vi "Drive Controller.vi"(8 "error in":errorcluster) -> ()   [LabVIEW 2018]
doc: "This VI executes continuously carrying out the current operation and responding to updates or new operation requests. It will often contain the timing or control code that is difficult to place directly in TeleOp. This VI generally opens all sensors and motors and isolates the rest of the robot code from knowing implementation details of how the operations are carried out."
uses:
  <vilib>/Rock Robotics/WPI/Framework/Completion Status.ctl
  Drive Setpoints.ctl
  Drive Operations.ctl
  Support Code/Path Data.ctl
  Support Code/Availible Command systems for auto.ctl
  <vilib>/Rock Robotics/WPI/ThirdParty/REV Robotics/SPARK MAX/Typedef/Spark MAX Control Type.ctl
  <vilib>/Rock Robotics/WPI/RobotDrive/WPI_RobotDriveArcadeDrive_Standard(NoSaturation).vi
  <vilib>/Rock Robotics/Network Tables/NT Read Number.vi
  <vilib>/Rock Robotics/Network Tables/NT Write Number.vi
  <vilib>/Rock Robotics/Network Tables/NT Write Boolean.vi
  ADIS16448 IMU/ADIS16448_IMU.lvlib
panel:
  in  "Time Home":u32=700
  in  "Time 90":u32=1000
  in  "Time 180":u32=1000
  in  "Interactive Values":T1 {"Auto Path Data"."Commands"."System" items=["FLoating Intake"=2, "Carriage Intake"=1, "Elevator"=0]; "Auto Path Data"."Commands"."System Selection" items=["FLoating Intake"=2, "Carriage Intake"=1, "Elevator"=0]}
  in  "Buttons":cluster{"Execute Cmd":bool, "Abort Cmd":bool}
  out "Command Timing":cluster{"Start Time (ms)":u32, "Iterations":i32}
  out "Status":T5
  out "Setpoints":T6(graph)
  out "Current\nCmd":string
  # "Tip: The graph shows the motor setpoints. It may also be helpful to observe inputs and sensor values.\nYou may also want to display tuning or debugging controls."
  # "Interactive Command: You may fill in the settings for a command\nand schedule it with the Execute button. You can observe and abort\nany command while fine tuning the code for the controller."
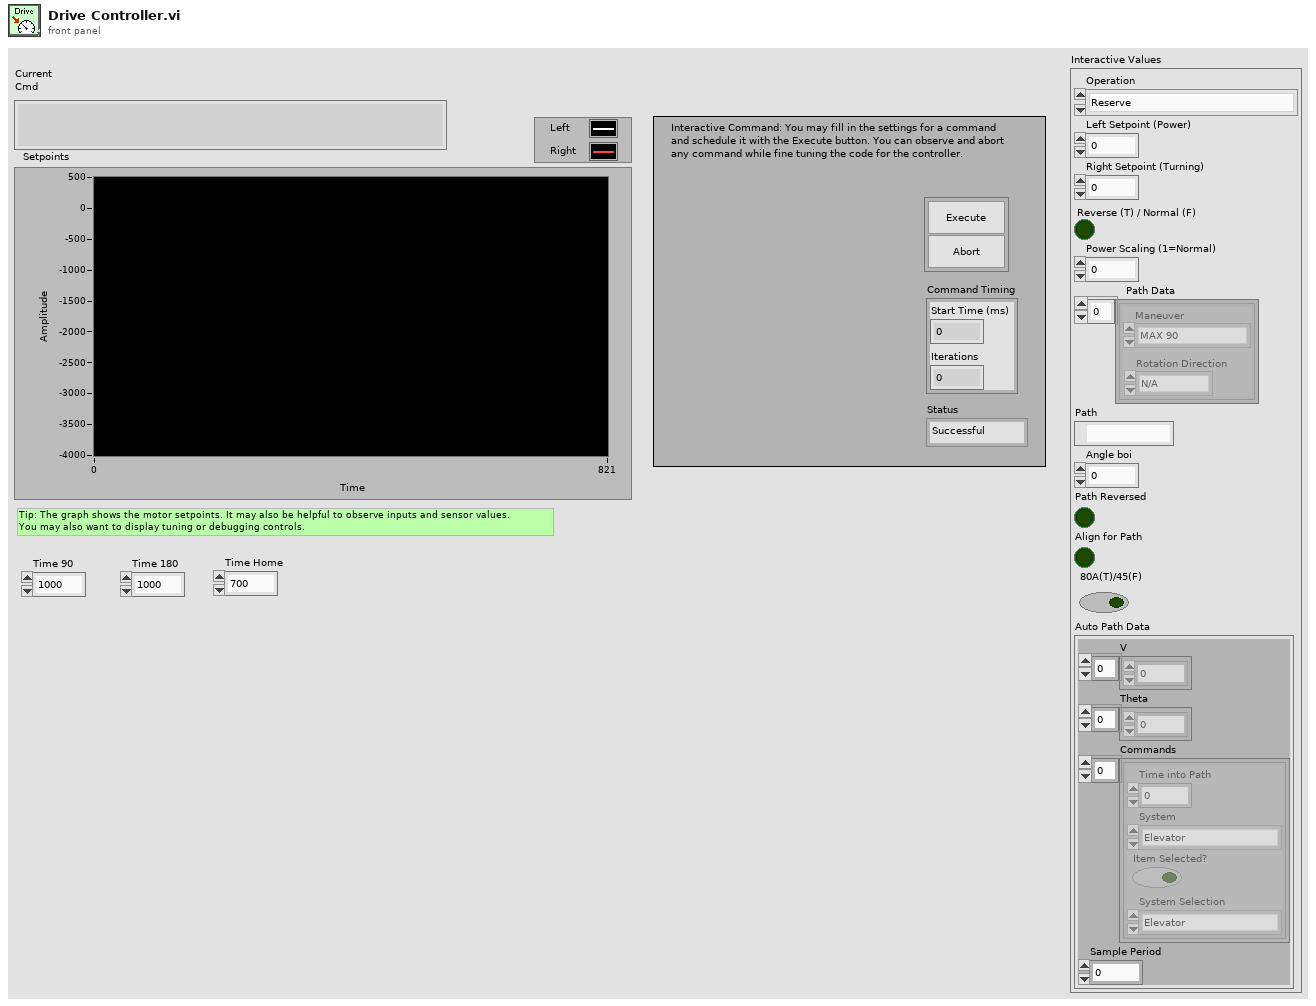
[diagram p1: front panel]
types:
  T1 = typedef "Drive Setpoints.ctl" = cluster{"Operation":T2, "Left Setpoint (Power)":dbl, "Right Setpoint (Turning)":dbl, "Reverse (T) / Normal (F)":bool, "Power Scaling (1=Normal) ":dbl, "Path Data":T3, "Path":path, "Angle boi":dbl, "Path Reversed":bool, "Align for Path":bool, "80A(T)/45(F)":bool, "Auto Path Data":cluster{"V":dbl[], "Theta":dbl[], "Commands":cluster{"Time into Path":dbl, "System":T4, "Item Selected?":bool, "System Selection":T4}[], "Sample Period":dbl}}
  T2 = typedef "Drive Operations.ctl" = enum16{"Reserve", "Read Current", "Immediate", "J-Turn", "Play Back From Log", "Auto-Align"}
  T3 = typedef "Path Data.ctl" = cluster{"Maneuver":enum16{"MAX 90", "MAX 180", "Turn to Home", "Turn to Rocket", "Auto-Align", "Turn to ..."}, "Rotation Direction":enum16{"N/A", "Right", "Left"}}[]
  T4 = typedef "Availible Command systems for auto.ctl" = u16
  T5 = typedef "Completion Status.ctl" = enum16{"Successful", "Aborted", "Incomplete"}
  T6 = cluster{"Left Setpoint":dbl, "Right Setpoint":dbl}
  T7 = cluster{"P Gain":dbl, "I Gain":dbl, "D Gain":dbl, "F Gain":dbl, "I Zone":dbl, "Min Output":dbl, "Max Output":dbl}
  T8 = typedef "WPI_MotorControlDeviceRef.ctl" = cluster{"DeviceStatus":errorcluster, "Type":T9, "PWM":cluster{"PWM Channel":T10, "DeadBand":T11}, "CAN":cluster{"Device Number":u8, "SetOutput VI Ref":variant, "GetOutput VI Ref":variant, "Enable VI Ref":variant, "Disable VI Ref":variant, "Data":variant}, "Invert":bool, "DIO PWM":cluster{"PWM \"Enable\" Channel":T10, "DIOChannel":T12, "PWM Rate":dbl}}
  T9 = typedef "WPI_MotorControlType.ctl" = enum16{"PWM", "CAN", "DIO PWM"}
  T10 = typedef "FPGA_DIOPWMChannel.ctl" = enum8{"PWM 0", "PWM 1", "PWM 2", "PWM 3", "PWM 4", "PWM 5", "PWM 6", "PWM 7", "PWM 8", "PWM 9", "PWM MXP 0", "PWM MXP 1", "PWM MXP 2", "PWM MXP 3", "PWM MXP 4", "PWM MXP 5", "PWM MXP 6", "PWM MXP 7", "PWM MXP 8", "PWM MXP 9", "Invalid"}
  T11 = typedef "WPI_PWMDeadband.ctl" = cluster{"Name":string, "maxPositivePwm":i32, "minPositivePwm":i32, "centerPwm":i32, "maxNegativePwm":i32, "minNegativePwm":i32, "angularRange":u16}
  T12 = typedef "FPGA_DIOChannel.ctl" = enum8{"DIO 0", "DIO 1", "DIO 2", "DIO 3", "DIO 4", "DIO 5", "DIO 6", "DIO 7", "DIO 8", "DIO 9", "DIO MXP 0", "DIO MXP 1", "DIO MXP 2", "DIO MXP 3", "DIO MXP 4", "DIO MXP 5", "DIO MXP 6", "DIO MXP 7", "DIO MXP 8", "DIO MXP 9", "DIO MXP 10", "DIO MXP 11", "DIO MXP 12", "DIO MXP 13", "DIO MXP 14", "DIO MXP 15", "SPI Port CS1", "SPI Port CS2", "SPI Port CS3", "SPI Port MISO", "SPI Port MOSI", "Invalid"}
  T13 = typedef "WPI_RobotDriveDevRef.ctl" = cluster{"DevStatus":errorcluster, "Motors[]":T8[], "Square Inputs":bool, "Max Output":dbl}
  T14 = typedef "ADIS16448_IMU.lvlib/ADI_IMU_ADIS16448_IMUDevRef.ctl" = cluster{"DevStatus":errorcluster, "Handle":i32, "SPI Bus":T15, "Device Found":bool, "Device Ready":bool, "Yaw Axis":enum16{"X", "Y", "Z"}, "AHRS Algorithm":enum16{"Complementary", "Madgwick"}, "Serial":u16, "Lot ID 2":u16, "Lot ID 1":u16, "Bytes Per Sample":u16, "Calibrate On Open?":bool}
  T15 = typedef "spi_bus.ctl" = enum16{"SPI On-Board, CS0", "SPI On-Board, CS1", "SPI On-Board, CS2", "SPI On-Board, CS3", "SPI MXP", "Invalid"}
  T16 = typedef "Command Status Info.ctl" = cluster{"Name":string, "Status":T5, "notifier out":T17}
  T17 = typedef "Completion Notifier.ctl" = refnum<notifier>
  T18 = cluster{"SubSystem Data":T1, cluster{"Start Time (ms)":u32, "Iterations":i32}, cluster{"Command Info":T16, "Description":string, "Default Command":T1, "queue out":refnum<queue>, "Subsystem Name":string}}
  T19 = enum16{"MAX 90", "MAX 180", "Turn to Home", "Turn to Rocket", "Auto-Align"}
  T20 = cluster{"proportional gain (Kc)":dbl, "integral time (Ti, min)":dbl, "derivative time (Td, min)":dbl}
  T21 = cluster{"V":dbl[], "Theta":dbl[], "Commands":cluster{"Time into Path":dbl, "System":T4, "Item Selected?":bool, "System Selection":T4}[], "Sample Period":dbl}
  T22 = cluster{"Maneuver":enum16{"MAX 90", "MAX 180", "Turn to Home", "Turn to Rocket", "Auto-Align", "Turn to ..."}, "Rotation Direction":enum16{"N/A", "Right", "Left"}}
  T23 = enum16{"MAX 90", "MAX 180", "Turn to Home", "Turn to Rocket", "Auto-Align", "Turn to ..."}
  T24 = typedef "Spark MAX Control Type.ctl" = enum16{"Percent VBus", "Voltage", "Velocity", "Position", "Smart Motion", "Current", "Smart Velocity"}
  T25 = cluster{"Time into Path":dbl, "System":T4, "Item Selected?":bool, "System Selection":T4}[]
  T26 = cluster{"Don't move motors while reserved":dbl, "Don't move motors while reserved":dbl}
  T27 = cluster{"SubSystem Data":T1, cluster{"Start Time (ms)":u32, "Iterations":i32}, "Default Command Arguments":cluster{"Command Info":T16, "Description":string, "Default Command":T1, "queue out":refnum<queue>, "Subsystem Name":string}}
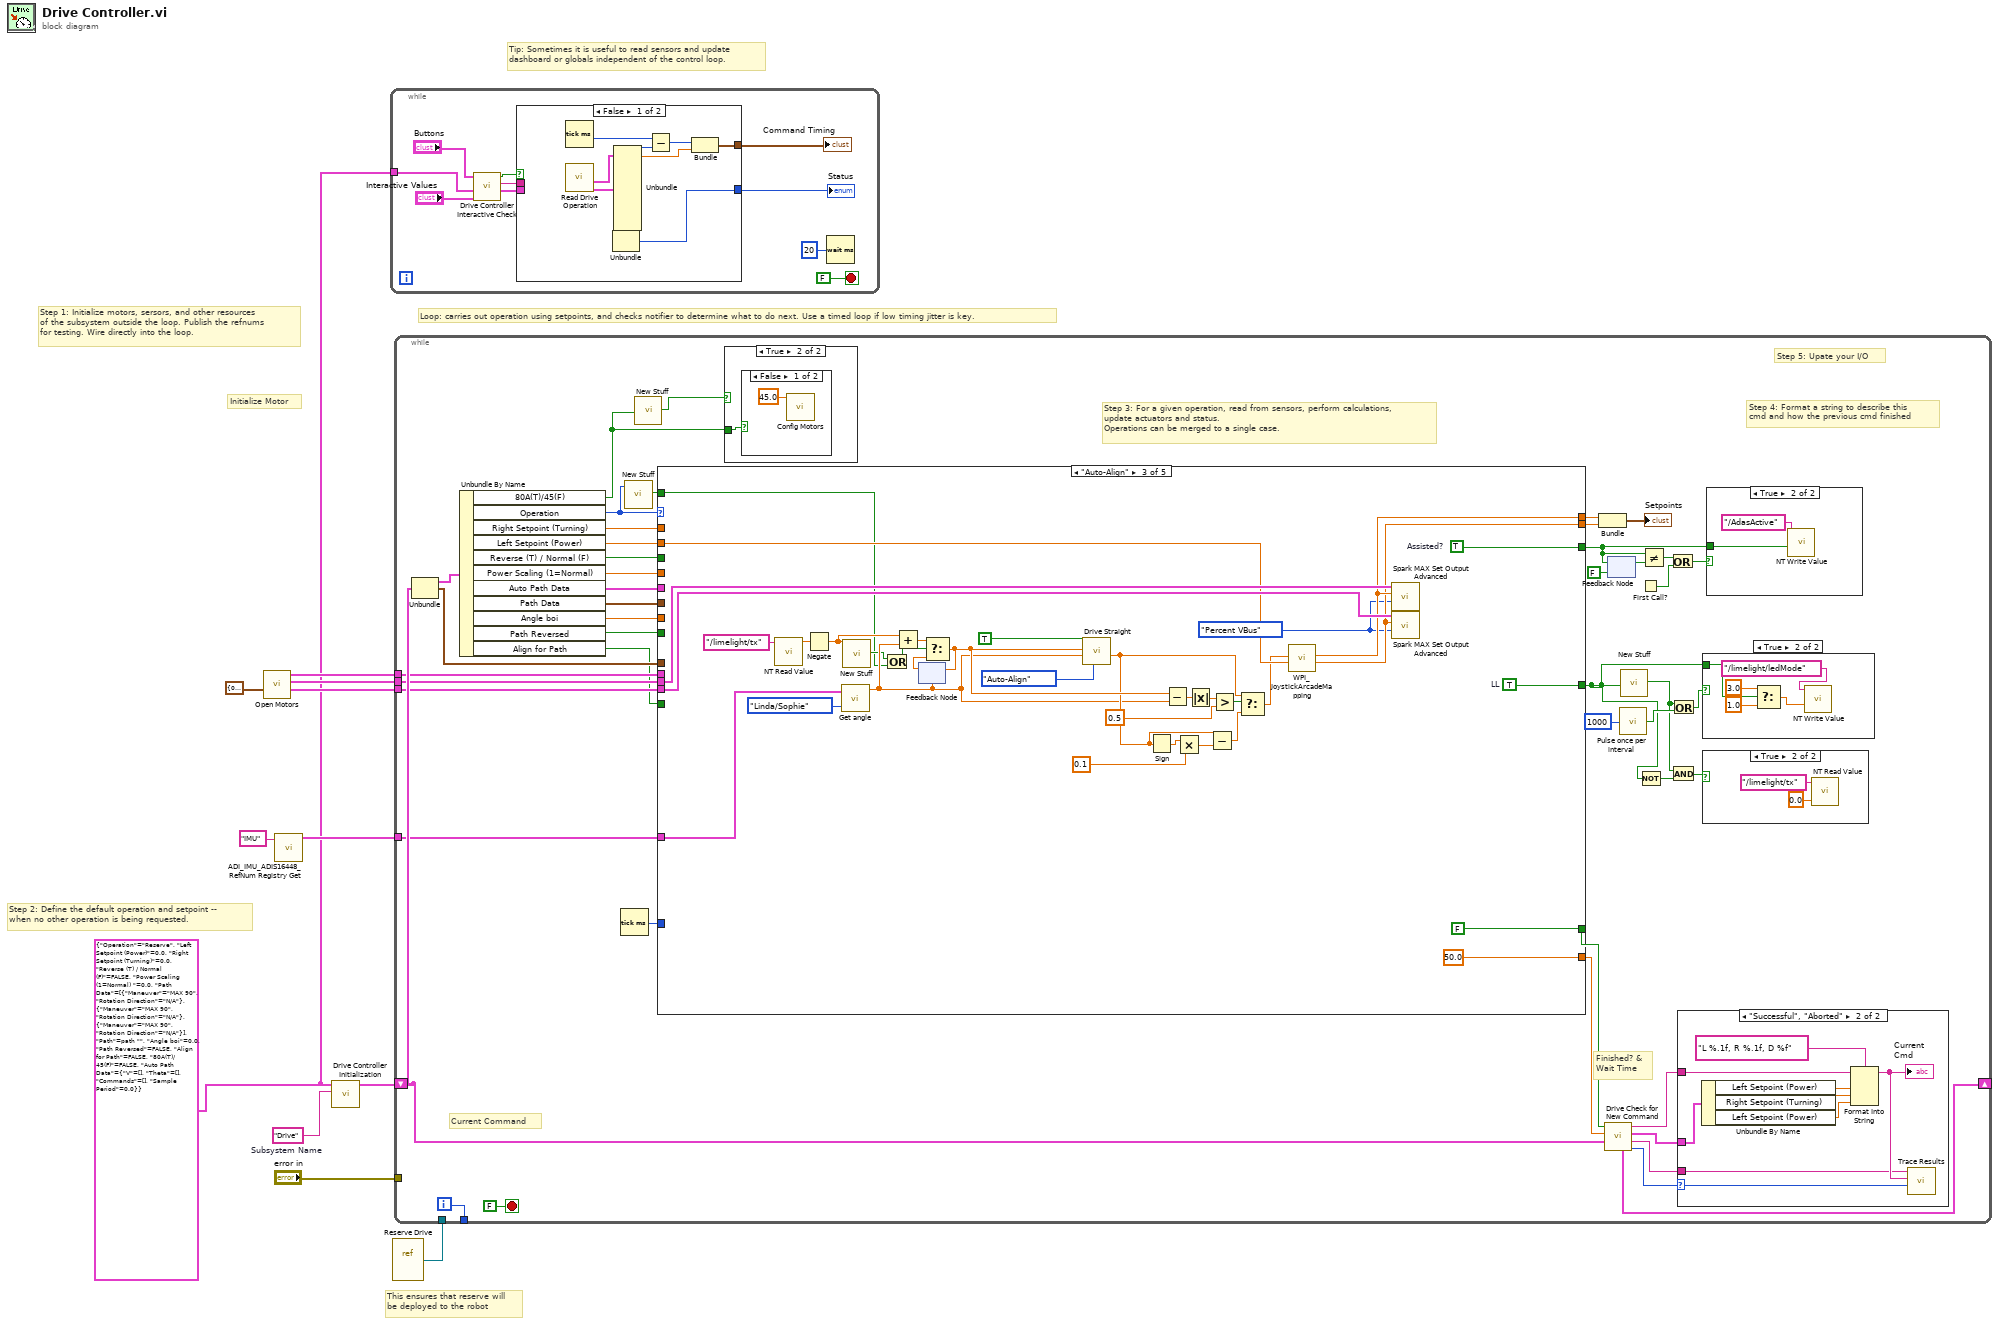
[diagram p0: block diagram]
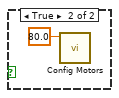
[diagram p4: hidden frame]
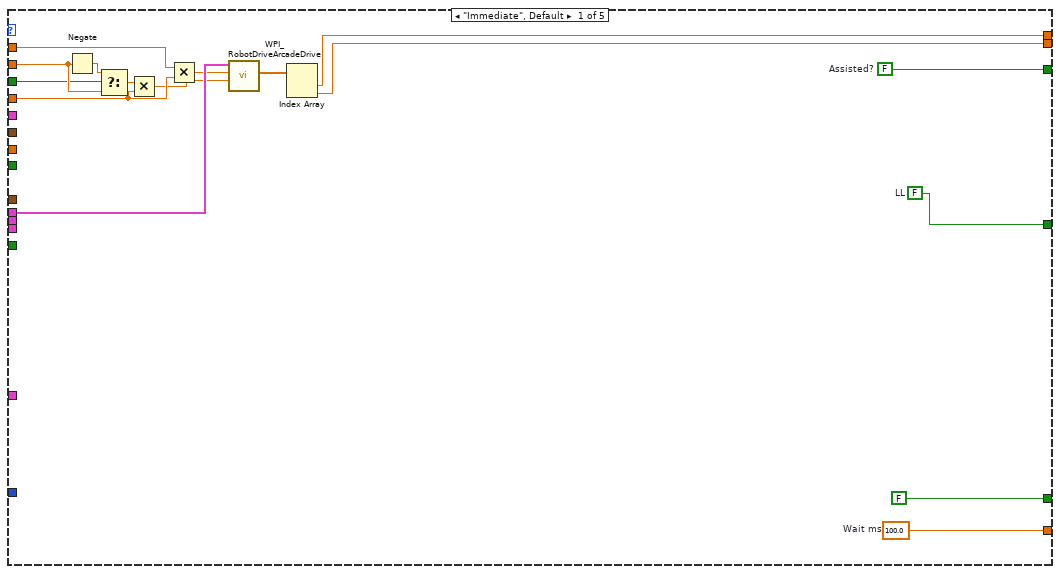
[diagram p6: hidden frame]
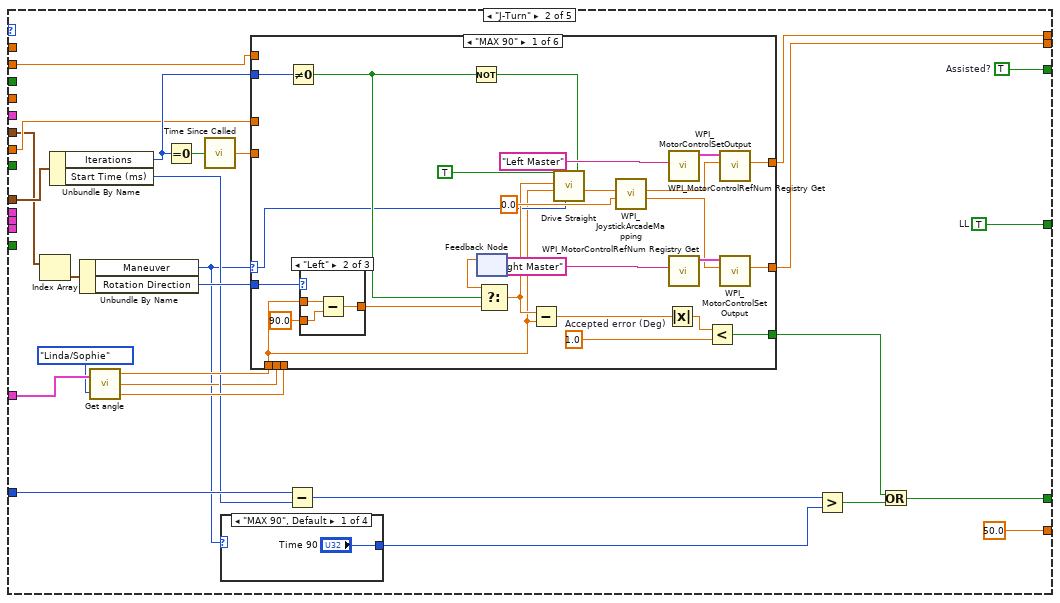
[diagram p7: hidden frame]
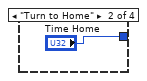
[diagram p8: hidden frame]
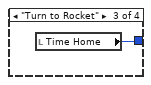
[diagram p9: hidden frame]
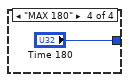
[diagram p10: hidden frame]
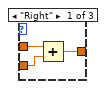
[diagram p11: hidden frame]
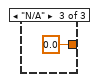
[diagram p12: hidden frame]
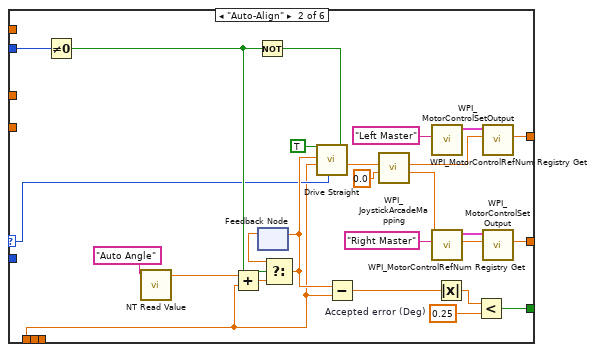
[diagram p13: hidden frame]
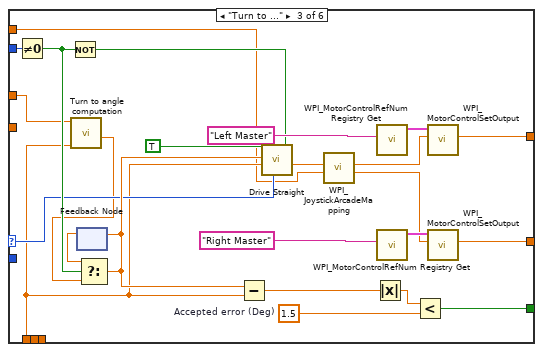
[diagram p14: hidden frame]
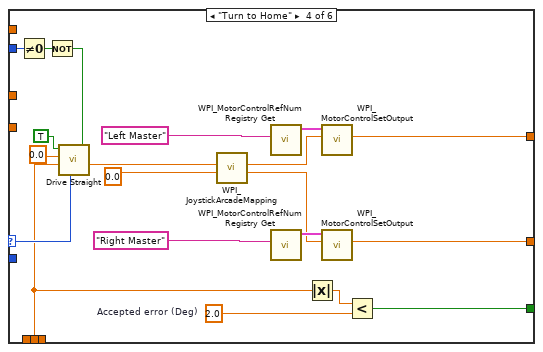
[diagram p15: hidden frame]
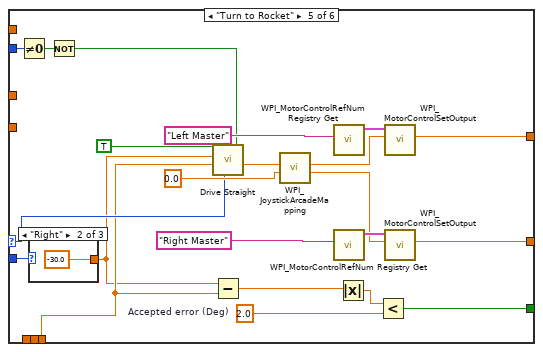
[diagram p16: hidden frame]
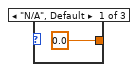
[diagram p17: hidden frame]
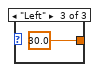
[diagram p18: hidden frame]
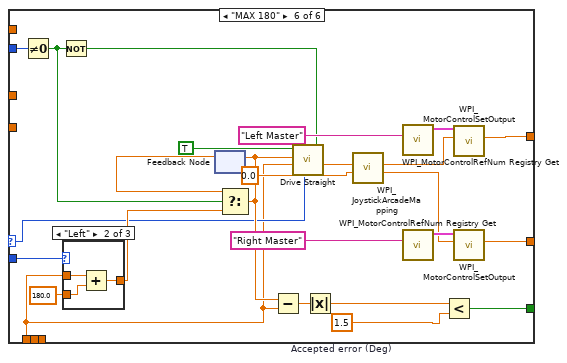
[diagram p19: hidden frame]
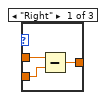
[diagram p20: hidden frame]
diagram:
  w1 = T1 {"Operation"=enum."Reserve", "Left Setpoint (Power)"=0.0, "Right Setpoint (Turning)"=0.0, "Reverse (T) / Normal (F)"=FALSE, "Power Scaling (1=Normal) "=0.0, "Path Data"=[{"Maneuver"=enum."MAX 90", "Rotation Direction"=enum."N/A"}, {"Maneuver"=enum."MAX 90", "Rotation Direction"=enum."N/A"}, {"Maneuver"=enum."MAX 90", "Rotation Direction"=enum."N/A"}], "Path"=path "", "Angle boi"=0.0, "Path Reversed"=FALSE, "Align for Path"=FALSE, "80A(T)/45(F)"=FALSE, "Auto Path Data"={"V"=[], "Theta"=[], "Commands"=[], "Sample Period"=0.0}} ("SubSystem Data")
  w11 = "Drive"  # Subsystem Name
  # "Initialize Motor"
  # "This ensures that reserve will\nbe deployed to the robot"
  # "Tip: Sometimes it is useful to read sensors and update\ndashboard or globals independent of the control loop."
  # "Step 2: Define the default operation and setpoint --\nwhen no other operation is being requested."
  # "Step 1: Initialize motors, sersors, and other resources\nof the subsystem outside the loop. Publish the refnums\nfor testing. Wire directly into the loop."
  # "Loop: carries out operation using setpoints, and checks notifier to determine what to do next. Use a timed loop if low timing jitter is key."
  n1 = call "Open Motors.vi"("PID Constants"=T7 {"P Gain"=0.00035, "I Gain"=5e-07, "D Gain"=0.0, "F Gain"=0.0002, "I Zone"=0.0, "Min Output"=-1.0, "Max Output"=1.0} ("PID Constants for Sparks")) -> ("Right"=w2:T8, "Left"=w3:T8, "WPI Robot"=w4:T13)  [unwired: 7 in, 1 out]
  n2 = call "ADI_IMU_ADIS16448_RefNum Registry Get.vi"("refnum name"="IMU") -> ("ADI IMU DevRef"=w6:T14)  [unwired: 9 in, 1 out]
  n3 = call "Drive Controller Initialization.vi"("Subsystem Name"=w11, "Default Command"=w1) -> ("Current Command"=w9:T18)  [unwired: 9 in]
  n4 = while {
    tunnel: w1 -> [w13]
    stop <- FALSE stop-if-true
    n5 = call "Drive Controller Interactive Check.vi"("Interactive Command In"="Interactive Values", "Default Command"=w13, "Buttons"="Buttons") -> ("Interactive Command Out"=w15:T1, "Trace String"=w16:string, "Schedule"=w17:bool)  [unwired: 6 in]
    n6 = case shown="False" w17 {
      tunnel: [w26 w34] -> w18
      tunnel: [w25 w30] -> w19
      tunnel: w16 -> [_ w32]
      tunnel: w15 -> [_ w31]
      frame False {
        n7 = Tick Count (ms)() -> (millisecond timer value=w29:u32)
        n8 = call "Read Drive Operation.vi"() -> ("Command Info"=w23:T16, "SubSystem Data"=w22:T1)  [unwired: 9 in, 1 out]
        n9 = Unbundle(w23) -> ("Status"=w26:T5)  [unwired: 2 out]
        n10 = Unbundle(w22) -> ("Operation"=w27:T2, "Left Setpoint (Power)"=w24:dbl)  [unwired: 10 out]
        n11 = Subtract(x=w29, y=w27) -> (x-y=w28:u32)
        n12 = Bundle(w28, "Left Setpoint (Power)"=w24) -> (w25:cluster{u32, "Left Setpoint (Power)":dbl})  [unwired: 1 in]
      }
      frame True {
        n13 = call "Drive Command Helper.vi"("Description"=w32, "SubSystem Data"=w31) -> ("Command Info Out"=w33:T16, "Command Timing"=w30:cluster{"Start Time (ms)":u32, "Iterations":i32})  [unwired: 7 in, 1 out]
        n14 = Unbundle(w33) -> ("Status"=w34:T5)  [unwired: 2 out]
      }
    }
    "Status" <- w18
    "Command Timing" <- w19
    n15 = Wait (ms)(milliseconds to wait=u32 20) -> ()  [unwired: 1 out]
  }
  n16 = vi-ref "Reserve Drive.vi"() -> (w8:refnum<vi>)
  n17 = while {
    shift-right: [w70] -> _
    shift-left: w9 -> [w63]
    tunnel: [w79] -> _
    tunnel: "error in" -> [_]
    tunnel: w8 -> [_]
    tunnel: w4 -> [w62]
    tunnel: w6 -> [w47]
    tunnel: w3 -> [w52]
    tunnel: w2 -> [w51]
    i -> [w79]
    stop <- FALSE stop-if-true
    # "Step 4: Format a string to describe this\ncmd and how the previous cmd finished"
    # "Step 5: Upate your I/O"
    # "Current Command"
    # "Finished? &\nWait Time"
    # "Step 3: For a given operation, read from sensors, perform calculations,\nupdate actuators and status.\nOperations can be merged to a single case."
    n18 = Unbundle(w63) -> ("SubSystem Data"=w75:T1, w64:cluster{"Start Time (ms)":u32, "Iterations":i32})  [unwired: 1 out]
    n19 = Unbundle By Name(w75) -> ("80A(T)/45(F)"=w40:bool, "Operation"=w50:T2, "Right Setpoint (Turning)"=w74:dbl, "Left Setpoint (Power)"=w73:dbl, "Reverse (T) / Normal (F)"=w61:bool, "Power Scaling (1=Normal)"=w60:dbl, "Auto Path Data"=w53:T21, "Path Data"=w39:T3, "Angle boi"=w48:dbl, "Path Reversed"=w46:bool, "Align for Path"=w45:bool)
    n20 = Tick Count (ms)() -> (millisecond timer value=w72:u32)
    n21 = call "New Stuff.vi"("Variant 2"=w50) -> ("x != y?"=w49:bool)  [unwired: 26 in]
    n22 = call "New Stuff.vi"("Variant 16"=w40) -> ("x != y?"=w41:bool)  [unwired: 26 in]
    n23 = case shown="\"Auto-Align\"" w50 {
      tunnel: [w106 50.0 ("Infinite") 50.0 ("Infinite") 20.0 ("Infinite") w364] -> w69
      tunnel: [FALSE ("ignore previous (F)") w128 FALSE ("ignore previous (F)") w349 FALSE ("ignore previous (F)")] -> w68
      tunnel: w64 -> [_ w130 _ w355 w363]
      tunnel: [w95 w125 w322 w346 w366] -> w77
      tunnel: [w94 w124 w321 w347 w366] -> w76
      tunnel: w74 -> [w98 _ _ w339 _]
      tunnel: w73 -> [w104 w112 w323 _ _]
      tunnel: w72 -> [_ w126 _ w354 _]
      tunnel: w62 -> [w101 _ _ _ w367]
      tunnel: w61 -> [w100 _ _ w345 _]
      tunnel: w60 -> [w99 _ _ _ _]
      tunnel: w47 -> [_ w123 w328 w352 w361]
      tunnel: [w97 w115 w327 TRUE ("Assisted?") w365] -> w59
      tunnel: w53 -> [_ _ _ w335 _]
      tunnel: w52 -> [_ _ w325 w337 _]
      tunnel: w51 -> [_ _ w324 w336 _]
      tunnel: w49 -> [_ _ w296 _ _]
      tunnel: w48 -> [_ w113 _ _ _]
      tunnel: w46 -> [_ _ _ w343 _]
      tunnel: w45 -> [_ _ _ w340 _]
      tunnel: [w91 w110 w320 w338 w358] -> w36
      tunnel: w39 -> [_ w109 _ _ _]
      frame "Immediate", Default {
        w91 = FALSE  # LL
        w97 = FALSE  # Assisted?
        w106 = 100.0  # Wait ms
        n24 = Negate(x=w104) -> (-x=w105:dbl)
        n25 = Select(t=w105, s=w100, f=w104) -> (s? t:f=w103:dbl)
        n26 = Multiply(x=w103, y=w99) -> (x*y=w93:dbl)
        n27 = Multiply(x=w98, y=w99) -> (x*y=w92:dbl)
        n28 = call-poly <vilib>:"WPI_RobotDriveArcadeDrive.vi"("Y axis value"=w93, "X axis value"=w92, "RobotDriveDevRef"=w101) -> ("Motor Values"=w96:dbl[])  [unwired: 6 in, 2 out]
        n29 = Index Array(array=w96) -> (element #1=w95:dbl, element #2=w94:dbl)  [unwired: 2 in]
      }
      frame "J-Turn" {
        w110 = TRUE  # LL
        w115 = TRUE  # Assisted?
        n30 = Index Array(array=w109) -> (element=w108:T22)  [unwired: 1 in]
        n31 = Unbundle By Name(w130) -> ("Iterations"=w118:i32, "Start Time (ms)"=w117:u32)
        n32 = Unbundle By Name(w108) -> ("Maneuver"=w107:T23, "Rotation Direction"=w132:enum16{"N/A", "Right", "Left"})
        n33 = call "Get angle.vi"("ADI IMU DevRef Out"=w123, "Robot"=enum16{"Linda/Sophie", "Mule"}."Linda/Sophie") -> ("Out"=w122:dbl, "Turn to Home"=w116:dbl, "Wraped Out"=w121:dbl)
        n34 = Equal To 0?(x=w118) -> (x = 0?=w131:bool)
        n35 = call "Time Since Called.vi"("Reset"=w131) -> ("Numeric"=w133:dbl)
        n36 = case shown="\"MAX 90\", Default" w107 {
          tunnel: ["Time 90" "Time Home" w136 "Time 180"] -> w120
          frame "MAX 90", Default {
          }
          frame "Turn to Home" {
          }
          frame "Turn to Rocket" {
            n37 = local read "Time Home"() -> (w136:u32)
          }
          frame "MAX 180" {
          }
        }
        n38 = case shown="\"MAX 90\"" w107 {
          selector: w107 -> [w140 w174 w199 w222 w243 w272]
          tunnel: [w142 w176 w201 w224 w245 w278] -> w119
          tunnel: w133 -> [_ _ _ _ _ _]
          tunnel: [w150 w184 w209 w230 w251 w269] -> w125
          tunnel: [w147 w181 w206 w227 w248 w266] -> w124
          tunnel: w132 -> [w138 _ _ _ w239 w264]
          tunnel: w118 -> [w141 w175 w200 w223 w244 w276]
          tunnel: w122 -> [w139 w170 w196 _ _ w265]
          tunnel: w121 -> [_ _ _ _ w241 _]
          tunnel: w116 -> [_ _ _ w221 _ _]
          tunnel: w113 -> [_ _ w198 _ _ _]
          tunnel: w112 -> [_ _ w195 _ _ _]
          frame "MAX 90" {
            w154 = 1.0  # Accepted error (Deg)
            n39 = Not Equal To 0?(x=w141) -> (x != 0?=w144:bool)
            n40 = case shown="\"Left\"" w138 {
              tunnel: 90.0 -> [w165 w168 _]
              tunnel: [w164 w167 0.0] -> w161
              tunnel: w139 -> [w163 w166 _]
              frame "Right" {
                n41 = Add(x=w163, y=w165) -> (x+y=w164:dbl)
              }
              frame "Left" {
                n42 = Subtract(x=w166, y=w168) -> (x-y=w167:dbl)
              }
              frame "N/A" {
              }
            }
            n43 = Not(x=w144) -> (.not. x?=w145:bool)
            n44 = feedback #1() -> (w160:dbl)  [unwired: 1 in]
            n45 = Select(t=w160, s=w144, f=w161) -> (s? t:f=w146:dbl)
            n46 = feedback-in #1(w146) -> ()
            n47 = Subtract(x=w146, y=w139) -> (x-y=w143:dbl)
            n48 = call "Drive Straight.vi"("reinitialize? (F)"=w145, "Maneuver"=w140, "Angle"=w139, "Angle to Get"=w146, "Enable?"=TRUE ("Drive Straight?")) -> ("Turn Setpoint"=w157:dbl)  [unwired: 4 in]
            n49 = call <vilib>:"WPI_JoystickArcadeMapping.vi"("Y axis value"=0.0, "X axis value"=w157) -> ("Right Motor Value"=w148:dbl, "Left Motor Value"=w152:dbl)  [unwired: 8 in]
            n50 = Absolute Value(x=w143) -> (abs(x)=w155:dbl)
            n51 = call <vilib>:"WPI_MotorControlRefNum Registry Get.vi"("refnum name"="Left Master") -> ("MotorControlDevRef"=w151:T8)  [unwired: 9 in, 1 out]
            n52 = call <vilib>:"WPI_MotorControlRefNum Registry Get.vi"("refnum name"="Right Master") -> ("MotorControlDevRef"=w149:T8)  [unwired: 9 in, 1 out]
            n53 = Less?(x=w155, y=w154) -> (x < y?=w142:bool)
            n54 = call <vilib>:"WPI_MotorControlSetOutput.vi"("Output"=w152, "MotorControlDevRef"=w151) -> ("Motor Output"=w150:dbl)  [unwired: 7 in, 2 out]
            n55 = call <vilib>:"WPI_MotorControlSetOutput.vi"("Output"=w148, "MotorControlDevRef"=w149) -> ("Motor Output"=w147:dbl)  [unwired: 7 in, 2 out]
          }
          frame "Auto-Align" {
            w188 = 0.25  # Accepted error (Deg)
            n56 = Not Equal To 0?(x=w175) -> (x != 0?=w178:bool)
            n57 = call-poly <vilib>:"NT Read Value.vi"("Name"="Auto Angle") -> ("Numeric"=w171:dbl)  [unwired: 9 in, 1 out]
            n58 = Add(x=w171, y=w170) -> (x+y=w172:dbl)
            n59 = Not(x=w178) -> (.not. x?=w179:bool)
            n60 = feedback #2() -> (w194:dbl)  [unwired: 1 in]
            n61 = Select(t=w194, s=w178, f=w172) -> (s? t:f=w180:dbl)
            n62 = feedback-in #2(w180) -> ()
            n63 = call "Drive Straight.vi"("reinitialize? (F)"=w179, "Maneuver"=w174, "Angle"=w170, "Angle to Get"=w180, "Enable?"=TRUE ("Drive Straight?")) -> ("Turn Setpoint"=w191:dbl)  [unwired: 4 in]
            n64 = Subtract(x=w180, y=w170) -> (x-y=w177:dbl)
            n65 = call <vilib>:"WPI_JoystickArcadeMapping.vi"("Y axis value"=0.0, "X axis value"=w191) -> ("Right Motor Value"=w182:dbl, "Left Motor Value"=w186:dbl)  [unwired: 8 in]
            n66 = call <vilib>:"WPI_MotorControlRefNum Registry Get.vi"("refnum name"="Left Master") -> ("MotorControlDevRef"=w185:T8)  [unwired: 9 in, 1 out]
            n67 = call <vilib>:"WPI_MotorControlRefNum Registry Get.vi"("refnum name"="Right Master") -> ("MotorControlDevRef"=w183:T8)  [unwired: 9 in, 1 out]
            n68 = Absolute Value(x=w177) -> (abs(x)=w189:dbl)
            n69 = Less?(x=w189, y=w188) -> (x < y?=w176:bool)
            n70 = call <vilib>:"WPI_MotorControlSetOutput.vi"("Output"=w186, "MotorControlDevRef"=w185) -> ("Motor Output"=w184:dbl)  [unwired: 7 in, 2 out]
            n71 = call <vilib>:"WPI_MotorControlSetOutput.vi"("Output"=w182, "MotorControlDevRef"=w183) -> ("Motor Output"=w181:dbl)  [unwired: 7 in, 2 out]
          }
          frame "Turn to ..." {
            w213 = 1.5  # Accepted error (Deg)
            n72 = Not Equal To 0?(x=w200) -> (x != 0?=w203:bool)
            n73 = Not(x=w203) -> (.not. x?=w204:bool)
            n74 = call "Turn to angle computation.vi"("Current Angle"=w196, "Angle To Get"=w198) -> ("Current Angle 2"=w197:dbl)  [unwired: 9 in]
            n75 = feedback #3() -> (w218:dbl)  [unwired: 1 in]
            n76 = Select(t=w218, s=w203, f=w197) -> (s? t:f=w205:dbl)
            n77 = feedback-in #3(w205) -> ()
            n78 = Subtract(x=w205, y=w196) -> (x-y=w202:dbl)
            n79 = call "Drive Straight.vi"("reinitialize? (F)"=w204, "Maneuver"=w199, "Angle"=w196, "Angle to Get"=w205, "Enable?"=TRUE ("Drive Straight?")) -> ("Turn Setpoint"=w215:dbl)  [unwired: 4 in]
            n80 = call <vilib>:"WPI_JoystickArcadeMapping.vi"("Y axis value"=w195, "X axis value"=w215) -> ("Right Motor Value"=w207:dbl, "Left Motor Value"=w211:dbl)  [unwired: 8 in]
            n81 = Absolute Value(x=w202) -> (abs(x)=w214:dbl)
            n82 = call <vilib>:"WPI_MotorControlRefNum Registry Get.vi"("refnum name"="Left Master") -> ("MotorControlDevRef"=w210:T8)  [unwired: 9 in, 1 out]
            n83 = call <vilib>:"WPI_MotorControlRefNum Registry Get.vi"("refnum name"="Right Master") -> ("MotorControlDevRef"=w208:T8)  [unwired: 9 in, 1 out]
            n84 = Less?(x=w214, y=w213) -> (x < y?=w201:bool)
            n85 = call <vilib>:"WPI_MotorControlSetOutput.vi"("Output"=w211, "MotorControlDevRef"=w210) -> ("Motor Output"=w209:dbl)  [unwired: 7 in, 2 out]
            n86 = call <vilib>:"WPI_MotorControlSetOutput.vi"("Output"=w207, "MotorControlDevRef"=w208) -> ("Motor Output"=w206:dbl)  [unwired: 7 in, 2 out]
          }
          frame "Turn to Home" {
            w233 = 2.0  # Accepted error (Deg)
            n87 = Not Equal To 0?(x=w223) -> (x != 0?=w225:bool)
            n88 = Not(x=w225) -> (.not. x?=w226:bool)
            n89 = call "Drive Straight.vi"("reinitialize? (F)"=w226, "Maneuver"=w222, "Angle"=w221, "Angle to Get"=0.0 ("Drive Setpoint"), "Enable?"=TRUE ("Drive Straight?")) -> ("Turn Setpoint"=w236:dbl)  [unwired: 4 in]
            n90 = call <vilib>:"WPI_JoystickArcadeMapping.vi"("Y axis value"=0.0, "X axis value"=w236) -> ("Right Motor Value"=w228:dbl, "Left Motor Value"=w232:dbl)  [unwired: 8 in]
            n91 = call <vilib>:"WPI_MotorControlRefNum Registry Get.vi"("refnum name"="Left Master") -> ("MotorControlDevRef"=w231:T8)  [unwired: 9 in, 1 out]
            n92 = call <vilib>:"WPI_MotorControlRefNum Registry Get.vi"("refnum name"="Right Master") -> ("MotorControlDevRef"=w229:T8)  [unwired: 9 in, 1 out]
            n93 = Absolute Value(x=w221) -> (abs(x)=w234:dbl)
            n94 = call <vilib>:"WPI_MotorControlSetOutput.vi"("Output"=w232, "MotorControlDevRef"=w231) -> ("Motor Output"=w230:dbl)  [unwired: 7 in, 2 out]
            n95 = call <vilib>:"WPI_MotorControlSetOutput.vi"("Output"=w228, "MotorControlDevRef"=w229) -> ("Motor Output"=w227:dbl)  [unwired: 7 in, 2 out]
            n96 = Less?(x=w234, y=w233) -> (x < y?=w224:bool)
          }
          frame "Turn to Rocket" {
            w255 = 2.0  # Accepted error (Deg)
            n97 = Not Equal To 0?(x=w244) -> (x != 0?=w246:bool)
            n98 = case shown="\"Right\"" w239 {
              tunnel: [0.0 -30.0 30.0] -> w240
              frame "N/A", Default {
              }
              frame "Right" {
              }
              frame "Left" {
              }
            }
            n99 = Not(x=w246) -> (.not. x?=w247:bool)
            n100 = call "Drive Straight.vi"("reinitialize? (F)"=w247, "Maneuver"=w243, "Angle"=w241, "Angle to Get"=w240, "Enable?"=TRUE ("Drive Straight?")) -> ("Turn Setpoint"=w258:dbl)  [unwired: 4 in]
            n101 = Subtract(x=w240, y=w241) -> (x-y=w242:dbl)
            n102 = call <vilib>:"WPI_JoystickArcadeMapping.vi"("Y axis value"=0.0, "X axis value"=w258) -> ("Right Motor Value"=w249:dbl, "Left Motor Value"=w253:dbl)  [unwired: 8 in]
            n103 = call <vilib>:"WPI_MotorControlRefNum Registry Get.vi"("refnum name"="Left Master") -> ("MotorControlDevRef"=w252:T8)  [unwired: 9 in, 1 out]
            n104 = call <vilib>:"WPI_MotorControlRefNum Registry Get.vi"("refnum name"="Right Master") -> ("MotorControlDevRef"=w250:T8)  [unwired: 9 in, 1 out]
            n105 = Absolute Value(x=w242) -> (abs(x)=w256:dbl)
            n106 = Less?(x=w256, y=w255) -> (x < y?=w245:bool)
            n107 = call <vilib>:"WPI_MotorControlSetOutput.vi"("Output"=w253, "MotorControlDevRef"=w252) -> ("Motor Output"=w251:dbl)  [unwired: 7 in, 2 out]
            n108 = call <vilib>:"WPI_MotorControlSetOutput.vi"("Output"=w249, "MotorControlDevRef"=w250) -> ("Motor Output"=w248:dbl)  [unwired: 7 in, 2 out]
          }
          frame "MAX 180" {
            w279 = 1.5  # Accepted error (Deg)
            n109 = Not Equal To 0?(x=w276) -> (x != 0?=w275:bool)
            n110 = Not(x=w275) -> (.not. x?=w274:bool)
            n111 = case shown="\"Left\"" w264 {
              tunnel: 180.0 -> [w291 w294 _]
              tunnel: [w290 w293 0.0] -> w287
              tunnel: w265 -> [w289 w292 _]
              frame "Right" {
                n112 = Subtract(x=w289, y=w291) -> (x-y=w290:dbl)
              }
              frame "Left" {
                n113 = Add(x=w292, y=w294) -> (x+y=w293:dbl)
              }
              frame "N/A" {
              }
            }
            n114 = feedback #4() -> (w286:dbl)  [unwired: 1 in]
            n115 = Select(t=w286, s=w275, f=w287) -> (s? t:f=w277:dbl)
            n116 = feedback-in #4(w277) -> ()
            n117 = Subtract(x=w277, y=w265) -> (x-y=w281:dbl)
            n118 = call "Drive Straight.vi"("reinitialize? (F)"=w274, "Maneuver"=w272, "Angle"=w265, "Angle to Get"=w277, "Enable?"=TRUE) -> ("Turn Setpoint"=w283:dbl)  [unwired: 4 in]
            n119 = Absolute Value(x=w281) -> (abs(x)=w280:dbl)
            n120 = call <vilib>:"WPI_JoystickArcadeMapping.vi"("Y axis value"=0.0, "X axis value"=w283) -> ("Right Motor Value"=w267:dbl, "Left Motor Value"=w270:dbl)  [unwired: 8 in]
            n121 = call <vilib>:"WPI_MotorControlRefNum Registry Get.vi"("refnum name"="Left Master") -> ("MotorControlDevRef"=w271:T8)  [unwired: 9 in, 1 out]
            n122 = call <vilib>:"WPI_MotorControlRefNum Registry Get.vi"("refnum name"="Right Master") -> ("MotorControlDevRef"=w268:T8)  [unwired: 9 in, 1 out]
            n123 = Less?(x=w280, y=w279) -> (x < y?=w278:bool)
            n124 = call <vilib>:"WPI_MotorControlSetOutput.vi"("Output"=w270, "MotorControlDevRef"=w271) -> ("Motor Output"=w269:dbl)  [unwired: 7 in, 2 out]
            n125 = call <vilib>:"WPI_MotorControlSetOutput.vi"("Output"=w267, "MotorControlDevRef"=w268) -> ("Motor Output"=w266:dbl)  [unwired: 7 in, 2 out]
          }
        }
        n126 = Subtract(x=w126, y=w117) -> (x-y=w129:u32)
        n127 = Greater?(x=w129, y=w120) -> (0:w111:bool)
        n128 = Or(x=w119, y=w111) -> (x .or. y?=w128:bool)
      }
      frame "Auto-Align" {
        w318 = Spark_MAX_Control_Type."Percent VBus" ("Control Mode")
        w320 = TRUE  # LL
        w327 = TRUE  # Assisted?
        n129 = call-poly <vilib>:"NT Read Value.vi"("Name"="/limelight/tx") -> ("Numeric"=w307:dbl)  [unwired: 9 in, 1 out]
        n130 = Negate(x=w307) -> (-x=w306:dbl)
        n131 = call "Get angle.vi"("ADI IMU DevRef Out"=w328, "Robot"=enum16{"Linda/Sophie", "Mule"}."Linda/Sophie") -> ("Out"=w299:dbl)  [unwired: 2 out]
        n132 = call "New Stuff.vi"("Variant"=w306) -> ("x != y?"=w297:bool)  [unwired: 26 in]
        n133 = Or(x=w297, y=w296) -> (x .or. y?=w298:bool)
        n134 = Add(x=w306, y=w299) -> (x+y=w314:dbl)
        n135 = feedback #5(w299) -> (w315:dbl)
        n136 = Select(t=w314, s=w298, f=w315) -> (s? t:f=w309:dbl)
        n137 = feedback-in #5(w309) -> ()
        n138 = call "Drive Straight.vi"("Maneuver"=T19."Auto-Align", "Angle"=w299, "Angle to Get"=w309, "Enable?"=TRUE ("Drive Straight?")) -> ("Turn Setpoint"=w302:dbl)  [unwired: 5 in]
        n139 = Sign(1:w302) -> (0:w304:dbl)
        n140 = Subtract(x=w309, y=w299) -> (x-y=w310:dbl)
        n141 = Multiply(x=w304, y=0.1) -> (x*y=w301:dbl)
        n142 = Absolute Value(x=w310) -> (abs(x)=w311:dbl)
        n143 = Subtract(x=w302, y=w301) -> (x-y=w300:dbl)
        n144 = Greater?(x=w311, y=0.5) -> (0:w312:bool)
        n145 = Select(t=w302, s=w312, f=w300) -> (s? t:f=w308:dbl)
        n146 = call <vilib>:"WPI_JoystickArcadeMapping.vi"("Y axis value"=w323, "X axis value"=w308) -> ("Right Motor Value"=w321:dbl, "Left Motor Value"=w322:dbl)  [unwired: 8 in]
        n147 = call <vilib>:"Spark MAX Set Output Advanced.vi"("Control Mode"=w318, "Setpoint"=w322, "MotorControlDevRef"=w325) -> ()  [unwired: 7 in, 2 out]
        n148 = call <vilib>:"Spark MAX Set Output Advanced.vi"("Control Mode"=w318, "Setpoint"=w321, "MotorControlDevRef"=w324) -> ()  [unwired: 7 in, 2 out]
      }
      frame "Play Back From Log" {
        w338 = TRUE  # LL
        w348 = Spark_MAX_Control_Type."Velocity" ("Control Mode")
        n149 = Unbundle By Name(w355) -> ("Iterations"=w330:i32)
        n150 = Unbundle(w335) -> ("V"=w334:dbl[], "Theta"=w333:dbl[], "Commands"=w332:T25, "Sample Period"=w331:dbl)
        n151 = call "Execute Path with commands.vi"("Iterations"=w330, "Sample Period"=w331, "Commands"=w332) -> ()
        n152 = call "Get angle.vi"("ADI IMU DevRef Out"=w352, "Robot"=enum16{"Linda/Sophie", "Mule"}."Linda/Sophie") -> ("Out"=w351:dbl)  [unwired: 2 out]
        n153 = call "Calculate Velocity Setpoints.vi"("Negated"=w345, "Front is Back"=FALSE, "Reversed"=w343, "Iterations"=w330, "Time"=w354, "Velocity Data"=w334, "Angular Data (Relative)"=w333, "f"=0.17, "Align?"=w340, "PID gains L/S 2"=T20 {"proportional gain (Kc)"=0.08, "integral time (Ti, min)"=0.0, "derivative time (Td, min)"=0.001}, "Enum"=enum16{"Vantage", "Mule", "Linda/Sophie"}."Linda/Sophie", "Angle To Get"=w339, "IMU Input"=w351) -> ("Left Setpoint"=w346:dbl, "Finished?"=w349:bool, "Right Setpoint"=w347:dbl)  [unwired: 3 in, 1 out]
        n154 = call <vilib>:"Spark MAX Set Output Advanced.vi"("Control Mode"=w348, "Setpoint"=w346, "MotorControlDevRef"=w337) -> ()  [unwired: 7 in, 2 out]
        n155 = call <vilib>:"Spark MAX Set Output Advanced.vi"("Control Mode"=w348, "Setpoint"=w347, "MotorControlDevRef"=w336) -> ()  [unwired: 7 in, 2 out]
      }
      frame "Reserve" {
        w358 = FALSE  # LL
        w365 = FALSE  # Assisted?
        # "If loop needs to poll sensors or other\nvalues, use a timeout value. -1 waits for\nnext command to be sent."
        n156 = Unbundle By Name(w363) -> ("Iterations"=w362:i32)
        n157 = call "Get angle.vi"("ADI IMU DevRef Out"=w361, "Robot"=enum16{"Linda/Sophie", "Mule"}."Linda/Sophie") -> ("Out"=w359:dbl)  [unwired: 2 out]
        n158 = case shown="1, Default" w362 {
          tunnel: w367 -> [_ w373]
          tunnel: [nan ("Don't move motors while reserved") w372] -> w366
          tunnel: [100.0 ("Infinite") w371] -> w364
          tunnel: w359 -> [_ _]
          frame 0 {
          }
          frame 1, Default {
            w371 = -1.0  # Infinite
            w372 = 0.0  # Don't move motors while reserved
            n159 = call <vilib>:"WPI_RobotDriveMotors.vi"("RightSpeed"=w372, "LeftSpeed"=w372, "RobotDriveDevRef"=w373) -> ()  [unwired: 1 in, 8 out]
          }
        }
      }
    }
    n160 = case shown="True" w41 {
      tunnel: w40 -> [_ w83]
      frame False {
      }
      frame True {
        n161 = case shown="False" w83 {
          frame False {
            n162 = call "Config Motors.vi"("Primay Current Limit (80A)"=45.0) -> ()  [unwired: 11 in]
          }
          frame True {
            n163 = call "Config Motors.vi"("Primay Current Limit (80A)"=80.0) -> ()  [unwired: 11 in]
          }
        }
      }
    }
    n164 = Bundle("Don't move motors while reserved"=w77, "Don't move motors while reserved"=w76) -> (→"Setpoints":T26)  [unwired: 1 in]
    n165 = call "Drive Check for New Command.vi"("input cluster"=w63, "Wait time (ms)"=w69, "Finished?"=w68) -> ("Completion"=w71:T5, "Subsystem Name"=w65:string, "Current Command"=w66:T1, "Initial Trace String"=w67:string, "Next Command"=w70:T27)  [unwired: 4 in]
    n166 = feedback #6(FALSE ("Assisted?")) -> (w58:bool)
    n167 = feedback-in #6(w59) -> ()
    n168 = call "Pulse once per interval.vi"("Time (ms)"=u32 1000) -> ("Boolean"=w43:bool)
    n169 = call "New Stuff.vi"("Variant 16"=w36) -> ("x != y?"=w37:bool)  [unwired: 26 in]
    n170 = First Call?() -> (First Call?: T/F=w56:bool)
    n171 = Not(x=w36) -> (.not. x?=w38:bool)
    n172 = Not Equal?(x=w59, y=w58) -> (x != y?=w55:bool)
    n173 = Or(x=w55, y=w56) -> (x .or. y?=w54:bool)
    n174 = Or(x=w37, y=w43) -> (x .or. y?=w44:bool)
    n175 = And(x=w37, y=w38) -> (x .and. y?=w35:bool)
    n176 = case shown="\"Successful\", \"Aborted\"" w71 {
      selector: w71 -> [_ w384]
      tunnel: w67 -> [_ w379]
      tunnel: w66 -> [_ w380]
      tunnel: w65 -> [_ w376]
      frame "Incomplete", Default {
        # "Continuing current command"
      }
      frame "Successful", "Aborted" {
        # "Report and setup for next command"
        n177 = Unbundle By Name(w380) -> ("Left Setpoint (Power)"=w382:dbl, "Right Setpoint (Turning)"=w383:dbl, "Left Setpoint (Power)"=w377:dbl)
        n178 = Format Into String(format string="L %.1f, R %.1f, D %f", initial string=w379, w382, w383, w377) -> (resulting string=w378:string)  [unwired: 1 in, 1 out]
        "Current\nCmd" <- w378
        n179 = call <vilib>:"Trace Results.vi"("Status of previous command"=w384, "Description"=w378, "Subsystem"=w376) -> ()  [unwired: 9 in]
      }
    }
    n180 = case shown="True" w44 {
      tunnel: w36 -> [_ w90]
      frame False {
      }
      frame True {
        n181 = Select(t=3.0, s=w90, f=1.0) -> (s? t:f=w87:dbl)
        n182 = call-poly <vilib>:"NT Write Value.vi"("Numeric"=w87, "Name"="/limelight/ledMode") -> ()  [unwired: 9 in, 1 out]
      }
    }
    n183 = case shown="True" w35 {
      frame False {
      }
      frame True {
        n184 = call-poly <vilib>:"NT Read Value.vi"("Default Value"=0.0, "Name"="/limelight/tx") -> ()  [unwired: 8 in, 2 out]
      }
    }
    n185 = case shown="True" w54 {
      tunnel: w59 -> [_ w374]
      frame False {
      }
      frame True {
        n186 = call-poly <vilib>:"NT Write Value.vi"("Boolean"=w374, "Name"="/AdasActive") -> ()  [unwired: 9 in, 1 out]
      }
    }
  }
